vi "11_DvDt_OFF.vi"(0 "file path (IN)":path, 1 "VCE":dbl, 5 "Project #":string, 7 "Request #":string, 9 "TEST #":string, 11 "error in (no error)":errorcluster) -> (4 "file path (OUT)":path, 6 "Dv/Dt (V/us)":dbl, 8 "DONE Dv/Dt OFF":bool, 10 "OFF Region":waveform(dbl)[](graph) caption="DvDt off (V/us)", 13 "Dv (V)":dbl, 14 "Dt (ns)":dbl, 15 "error out":errorcluster)   [LabVIEW 2020]
uses:
  <vilib>/Waveform/WDTOps.llb/WDT Waveform Duration DBL.vi
  <vilib>/Waveform/WDTOps.llb/WDT Get Waveform Subset DBL.vi
  <vilib>/measure/mascope.llb/Transition Measurements 1 chan.vi
  <vilib>/measure/NI_MAPro.lvlib
panel:
  in  "Decision ?":bool
  out "Cursor b : Channel 3":dbl
  out "Cursor a : Channel 3":dbl
  in  "Cursor b : Channel 3 \nrise edge tolerance":dbl=0.1
  in  "Cursor b : Channel 3\nrise edge number":i32=1 min=1
  in  "Cursor a : Channel 3 \nrise edge tolerance":dbl=0.1
  in  "Cursor a : Channel 3\nrise edge number":i32=1 min=1
  out "Dt (us)":dbl
  out "80% Vce":dbl
  out "50% Vce":dbl
  out "measurement info (CH3 Cursor a)":T1 {"ref levels"."ref units" items=["absolute", "relative"]; "ref levels"."high ref level" format="%.2p"; "ref levels"."low ref level" format="%.2p"; "ref levels"."mid ref level" format="%.2p"; "end time" format="%.6e"; "start time" format="%.6e"}
  out "measurement info (CH3 Cursor b)":T1 {"ref levels"."ref units" items=["absolute", "relative"]; "ref levels"."high ref level" format="%.2p"; "ref levels"."low ref level" format="%.2p"; "ref levels"."mid ref level" format="%.2p"; "end time" format="%.6e"; "start time" format="%.6e"}
  in  "reference  levels (CH1 2nd Cursor)":T2={"high ref level"=90.0, "mid ref level"=50.0, "low ref level"=10.0, "ref units"=1} {"ref units" items=["absolute", "percent"]; "high ref level" format="%0.2f"; "low ref level" format="%0.2f"; "mid ref level" format="%0.2f"}
  in  "reference  levels (CH1 1st Cursor)":T2={"high ref level"=90.0, "mid ref level"=50.0, "low ref level"=10.0, "ref units"=1} {"ref units" items=["absolute", "percent"]; "high ref level" format="%0.2f"; "low ref level" format="%0.2f"; "mid ref level" format="%0.2f"}
  out "Waveform Graph":waveform(dbl)[](graph)
  # "From 50% to 80% of Peak Voltage"
  # "Default = 1"
  # "Default = 1"
  # "Default = 0.1"
  # "Default = 0.1"
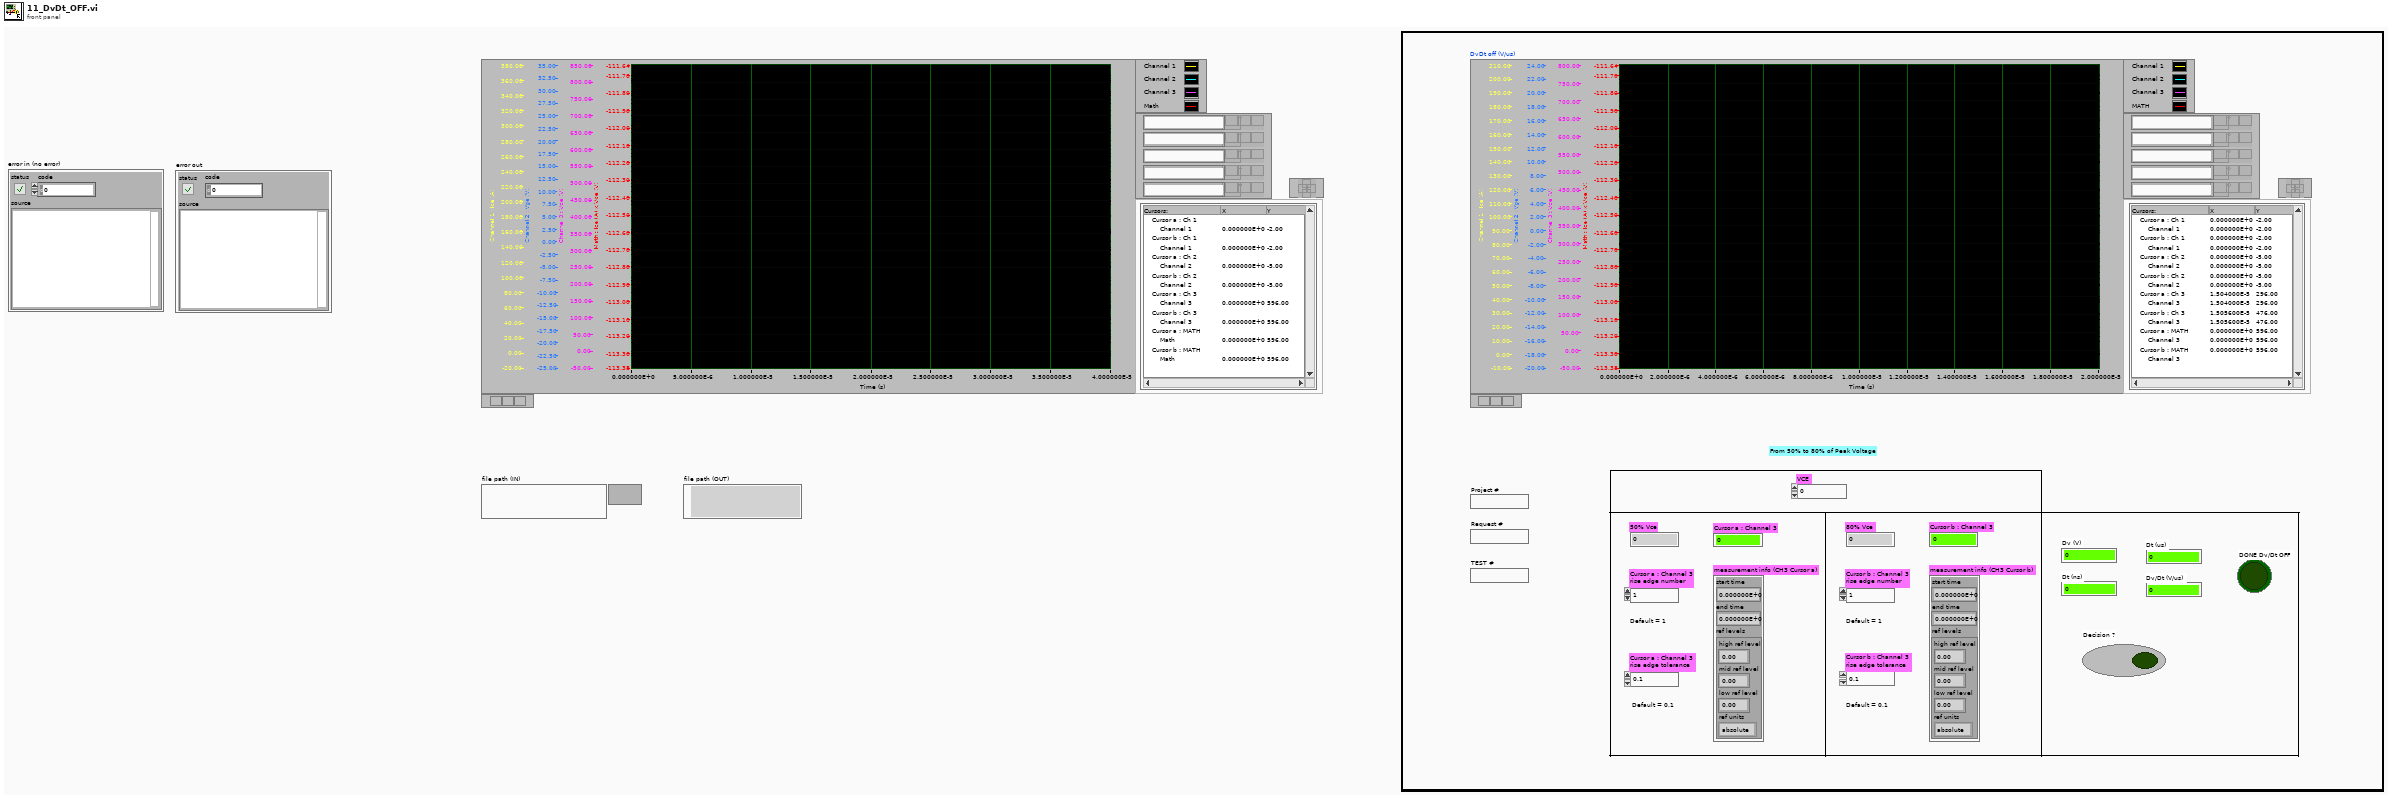
[diagram p1: front panel]
types:
  T1 = cluster{"start time":dbl, "end time":dbl, "ref levels":cluster{"high ref level":dbl, "mid ref level":dbl, "low ref level":dbl, "ref units":u16}}
  T2 = cluster{"high ref level":dbl, "mid ref level":dbl, "low ref level":dbl, "ref units":u16}
  T3 = enum32{"Invalid", "Standard", "Closed", "Hidden", "Minimized", "Maximized"}
  T4 = typedef "imagedata.ctl" = cluster{"image type":i32, "image depth":i32, "image":u8[], "mask":u8[], "colors":u32[], "Rectangle":cluster{"left":i16, "top":i16, "right":i16, "bottom":i16}}
diagram:
  w12 = 0.0 ("Dv (V)")
  w13 = errorcluster {"status"=FALSE, "code"=0, "source"=""} ("error out")
  w11 = FALSE ("DONE Tdon")
  w14 = waveform(dbl)[] [] ("Waveform Graph")
  n1 = local write "error out"(w13) -> ()
  n2 = local write "error in (no error)"(w13) -> ()
  n3 = local write "DONE Dv/Dt OFF"(w11) -> ()
  n4 = local write "Waveform Graph"(w14) -> ()
  n5 = local write "OFF Region"(w14) -> ()
  n6 = local write "Decision ?"(w11) -> ()
  n7 = local write "Cursor a : Channel 3 \nrise edge tolerance"(0.1 ("Cursor a : Channel 3 \nrise edge tolerance")) -> ()
  n8 = local write "Cursor a : Channel 3\nrise edge number"(1 ("Cursor a : Channel 3\nrise edge number")) -> ()
  n9 = local write "Cursor b : Channel 3 \nrise edge tolerance"(0.1 ("Cursor b : Channel 3 \nrise edge tolerance")) -> ()
  n10 = local write "Cursor b : Channel 3\nrise edge number"(1 ("Cursor b : Channel 3\nrise edge number")) -> ()
  n11 = local write "Dv (V)"(w12) -> ()
  n12 = local write "Dt (ns)"(w12) -> ()
  n13 = local write "Dt (us)"(w12) -> ()
  n14 = local write "Dv/Dt (V/us)"(w12) -> ()
  n15 = local write "Cursor a : Channel 3"(w12) -> ()
  n16 = local write "Cursor b : Channel 3"(w12) -> ()
  n17 = flat-sequence {
    tunnel: ["error in (no error)"] -> w6
    tunnel: ["file path (IN)"] -> w5
    tunnel: [w25] -> w9
    tunnel: [w24] -> w8
    tunnel: w6 -> [w23]
    tunnel: w5 -> [w22]
    tunnel: [w257] -> w10
    tunnel: w9 -> [w256]
    tunnel: w8 -> [w255]
    tunnel: [w255] -> w7
    tunnel: w10 -> [w270]
    tunnel: w7 -> [w271]
    frame #0 {
      n18 = control-ref of="This VI"() -> (w19:refnum<vi>)
      n19 = invoke class="VI" method="FP.Open"(reference=w19, error in="error in (no error)", "Activate"=TRUE ("Activate?"), "State"=T3."Maximized") -> (error out=w20:errorcluster)  [unwired: 1 in, 4 out]
      n20 = property class="VI"(reference=w19, error in=w20, "Front Panel.Closeable"=TRUE ("Front Panel Window:Closeable")) -> ()  [unwired: 2 out]
    }
    frame #1 {
      n21 = while {
        shift-right: [w30] -> w25
        shift-left: w23 -> [w32]
        tunnel: [w27] -> w24
        tunnel: w22 -> [w26]
        stop <- w29 stop-if-true
        n22 = flat-sequence {
          tunnel: [w58] -> w51
          tunnel: w32 -> [w63]
          tunnel: [w63] -> w31
          tunnel: w26 -> [w58]
          tunnel: w51 -> [w150]
          tunnel: [w79] -> w50
          tunnel: [w69] -> w49
          tunnel: [w65] -> w48
          tunnel: w31 -> [w156]
          tunnel: w50 -> [w199]
          tunnel: [w180] -> w47
          tunnel: w49 -> [w192]
          tunnel: [w192] -> w46
          tunnel: [w170] -> w45
          tunnel: [w169] -> w44
          tunnel: [w179] -> w43
          tunnel: [w178] -> w42
          tunnel: w48 -> [w177]
          tunnel: w47 -> [w226]
          tunnel: [w227] -> w41
          tunnel: w46 -> [w230]
          tunnel: [w230] -> w40
          tunnel: w45 -> [w229]
          tunnel: [w229] -> w39
          tunnel: w44 -> [w228]
          tunnel: [w228] -> w38
          tunnel: w43 -> [w220]
          tunnel: [w220] -> w37
          tunnel: w42 -> [w221]
          tunnel: [w221] -> w36
          tunnel: w41 -> [w231]
          tunnel: w40 -> [w244]
          tunnel: [w244] -> w35
          tunnel: w39 -> [w238]
          tunnel: w38 -> [w239]
          tunnel: w37 -> [w237]
          tunnel: w36 -> [w236]
          tunnel: [w231] -> w34
          tunnel: w35 -> [w249]
          tunnel: w34 -> [w251]
          tunnel: [w250] -> w33
          tunnel: [w249] -> w27
          frame #0 {
            w61 = 0.0 ("Dv (V)")
            w62 = FALSE ("DONE Tdon")
            w60 = waveform(dbl)[] [] ("Waveform Graph")
            n23 = local write "DONE Dv/Dt OFF"(w62) -> ()
            n24 = local write "Dv (V)"(w61) -> ()
            n25 = local write "Dt (ns)"(w61) -> ()
            n26 = local write "Dt (us)"(w61) -> ()
            n27 = local write "Dv/Dt (V/us)"(w61) -> ()
            n28 = local write "Decision ?"(w62) -> ()
            n29 = Wait (ms)(milliseconds to wait=u32 200) -> ()  [unwired: 1 out]
            n30 = local write "Cursor a : Channel 3"(w61) -> ()
            n31 = local write "Cursor b : Channel 3"(w61) -> ()
            n32 = local write "Waveform Graph"(w60) -> ()
            n33 = local write "OFF Region"(w60) -> ()
          }
          frame #1 {
            w64 = 0.0 ("start samples/time")
            w131 = u16 1 items=["Samples", "Relative Time"] ("start/duration format")
            w142 = u16 1 items=["Samples", "Relative Time"] ("start/duration format")
            w143 = u16 1 items=["Samples", "Relative Time"] ("start/duration format")
            # "Channel 1"
            # "Channel 3"
            # "Channel 2"
            # "dt"
            # "Ch2"
            # "Ch1"
            n34 = call "3_ReadDatatoWaveform.vi"("error in (no error)"=w156, "file path (IN)"=w150) -> ("error out"=w125:errorcluster, "Waveform Graph"=→"Waveform Graph":waveform(dbl)[], "file path (OUT)"=w69:path, "dt"=w151:dbl, "Ch 2 Data"=w148:dbl[], "Ch 3 Data"=w152:dbl[], "Ch 1 Data"=w149:dbl[])  [unwired: 3 in]
            n35 = To Time Stamp(1:0.0 ("number")) -> (0:w153:timestamp)
            n36 = disable-structure shown="Enabled" {
              disable-tunnel: w153 -> [w160 _]
              disable-tunnel: w151 -> [w159 _]
              disable-tunnel: w149 -> [w158 _]
              disable-tunnel: [w157 _] -> w130
              frame Enabled {
                # "Channel 1"
                n37 = Bundle By Name("Y"=w158, "dt"=w159, "t0"=w160) -> (w157:waveform(dbl))  [unwired: 1 in]
              }
              frame Disabled {
              }
            }
            n38 = disable-structure shown="Enabled" {
              disable-tunnel: w153 -> [w164 _]
              disable-tunnel: w151 -> [w163 _]
              disable-tunnel: w148 -> [w162 _]
              disable-tunnel: [w161 _] -> w129
              frame Enabled {
                # "Channel 2"
                n39 = Bundle By Name("Y"=w162, "dt"=w163, "t0"=w164) -> (w161:waveform(dbl))  [unwired: 1 in]
              }
              frame Disabled {
              }
            }
            n40 = disable-structure shown="Enabled" {
              disable-tunnel: w153 -> [w168 _]
              disable-tunnel: w151 -> [w167 _]
              disable-tunnel: w152 -> [w166 _]
              disable-tunnel: [w165 _] -> w128
              frame Enabled {
                # "Channel 3"
                n41 = Bundle By Name("Y"=w166, "dt"=w167, "t0"=w168) -> (w165:waveform(dbl))  [unwired: 1 in]
              }
              frame Disabled {
              }
            }
            n42 = call-poly <vilib>:"Waveform Duration.vi"("error in (no error)"=w125, "waveform in"=w128) -> ("error out"=w136:errorcluster, "duration"=w133:dbl, "waveform out"=w135:waveform(dbl))  [unwired: 7 in]
            n43 = call-poly <vilib>:"Waveform Duration.vi"("error in (no error)"=w125, "waveform in"=w129) -> ("error out"=w137:errorcluster, "duration"=w140:dbl, "waveform out"=w138:waveform(dbl))  [unwired: 7 in]
            n44 = call-poly <vilib>:"Waveform Duration.vi"("error in (no error)"=w125, "waveform in"=w130) -> ("error out"=w147:errorcluster, "duration"=w144:dbl, "waveform out"=w146:waveform(dbl))  [unwired: 7 in]
            n45 = Divide(x=w133, y=2.0) -> (x/y=w132:dbl)
            n46 = Divide(x=w140, y=2.0) -> (x/y=w141:dbl)
            n47 = Divide(x=w144, y=2.0) -> (x/y=w126:dbl)
            n48 = call-poly <vilib>:"Get Waveform Subset.vi"("start/duration format"=w131, "error in (no error)"=w136, "duration"=w132, "start samples/time"=w64, "waveform in"=w135) -> ("error out"=w122:errorcluster, "waveform out"=w65:waveform(dbl))  [unwired: 1 in, 2 out]
            n49 = call-poly <vilib>:"Get Waveform Subset.vi"("start/duration format"=w142, "error in (no error)"=w137, "duration"=w141, "start samples/time"=w64, "waveform in"=w138) -> ("error out"=w123:errorcluster, "waveform out"=w81:waveform(dbl))  [unwired: 1 in, 2 out]
            n50 = call-poly <vilib>:"Get Waveform Subset.vi"("start/duration format"=w143, "error in (no error)"=w147, "duration"=w126, "start samples/time"=w64, "waveform in"=w146) -> ("error out"=w124:errorcluster, "waveform out"=w80:waveform(dbl))  [unwired: 1 in, 2 out]
            n51 = Build Array(w80, w81, w65) -> (→"OFF Region":waveform(dbl)[])
            n52 = Merge Errors(w124, w123, w122) -> (w77:errorcluster)
            n53 = property on="OFF Region" class="WFGraph (strict)"(error in=w77) -> (error out=w76:errorcluster, "Width"=w75:u32)  [unwired: 1 in, 1 out]
            n54 = property on="OFF Region" class="WFGraph (strict)"(error in=w76, "Caption.Justify"=enum16{"Left", "Center", "Right"}."Left" ("Caption.Justification"), "Caption.Width"=w75, "Caption.FontBold"=TRUE ("Caption.Font:Bold"), "Caption.FontColor"=u32 16860 ("Caption.Font:Color"), "Caption.FontSize"=u32 24 ("Caption.Font:Size"), "Caption.Text"="DvDt off (V/us)") -> (error out=w71:errorcluster)  [unwired: 1 in, 1 out]
            n55 = property on="OFF Region" class="WFGraph (strict)"(error in=w71, "XScale.Offset"=w64) -> (error out=w105:errorcluster)  [unwired: 1 in, 1 out]
            n56 = property on="OFF Region" class="WFGraph (strict)"(error in=w105, "Active Cursor"=u32 0, "Cursor.Cursor X"=0.0 ("Cursor.Cursor Position:Cursor X"), "Cursor.Cursor Y"=0.0 ("Cursor.Cursor Position:Cursor Y"), "Cursor.Visible"=FALSE) -> (error out=w104:errorcluster)  [unwired: 1 in, 1 out]
            n57 = property on="OFF Region" class="WFGraph (strict)"(error in=w104, "Active Cursor"=u32 1, "Cursor.Cursor X"=0.0 ("Cursor.Cursor Position:Cursor X"), "Cursor.Cursor Y"=0.0 ("Cursor.Cursor Position:Cursor Y"), "Cursor.Visible"=FALSE) -> (error out=w103:errorcluster)  [unwired: 1 in, 1 out]
            n58 = property on="OFF Region" class="WFGraph (strict)"(error in=w103, "Active Cursor"=u32 2, "Cursor.Cursor X"=0.0 ("Cursor.Cursor Position:Cursor X"), "Cursor.Cursor Y"=0.0 ("Cursor.Cursor Position:Cursor Y"), "Cursor.Visible"=FALSE) -> (error out=w102:errorcluster)  [unwired: 1 in, 1 out]
            n59 = property on="OFF Region" class="WFGraph (strict)"(error in=w102, "Active Cursor"=u32 3, "Cursor.Cursor X"=0.0 ("Cursor.Cursor Position:Cursor X"), "Cursor.Cursor Y"=0.0 ("Cursor.Cursor Position:Cursor Y"), "Cursor.Visible"=FALSE) -> (error out=w85:errorcluster)  [unwired: 1 in, 1 out]
            n60 = property on="OFF Region" class="WFGraph (strict)"(error in=w85, "Active Cursor"=u32 4, "Cursor.Cursor X"=0.0 ("Cursor.Cursor Position:Cursor X"), "Cursor.Cursor Y"=0.0 ("Cursor.Cursor Position:Cursor Y"), "Cursor.Visible"=FALSE) -> (error out=w84:errorcluster)  [unwired: 1 in, 1 out]
            n61 = property on="OFF Region" class="WFGraph (strict)"(error in=w84, "Active Cursor"=u32 5, "Cursor.Cursor X"=0.0 ("Cursor.Cursor Position:Cursor X"), "Cursor.Cursor Y"=0.0 ("Cursor.Cursor Position:Cursor Y"), "Cursor.Visible"=FALSE) -> (error out=w83:errorcluster)  [unwired: 1 in, 1 out]
            n62 = property on="OFF Region" class="WFGraph (strict)"(error in=w83, "Active Cursor"=u32 6, "Cursor.Cursor X"=0.0 ("Cursor.Cursor Position:Cursor X"), "Cursor.Cursor Y"=0.0 ("Cursor.Cursor Position:Cursor Y"), "Cursor.Visible"=FALSE) -> (error out=w82:errorcluster)  [unwired: 1 in, 1 out]
            n63 = property on="OFF Region" class="WFGraph (strict)"(error in=w82, "Active Cursor"=u32 7, "Cursor.Cursor X"=0.0 ("Cursor.Cursor Position:Cursor X"), "Cursor.Cursor Y"=0.0 ("Cursor.Cursor Position:Cursor Y"), "Cursor.Visible"=FALSE) -> (error out=w79:errorcluster)  [unwired: 1 in, 1 out]
            n64 = call <vilib>:"Beep.vi"("use system alert? (T)"=FALSE, "duration (msec)"=u32 200, "frequency (Hz)"=u32 2000) -> ()  [unwired: 9 in]
          }
          frame #2 {
            w212 = u16 1 items=["falling", "rising"] ("polarity (rising)")
            w213 = u16 1 items=["falling", "rising"] ("polarity (rising)")
            # "XPOS"
            # "YPOS"
            # "Cursor a : Channel 1"
            # "Cursor b : Channel 1"
            # "Cursor b : Channel 1"
            # "Cursor a : Channel 1"
            # "Cursor b : Channel 1"
            # "Cursor a : Channel 3"
            # "Cursor b : Channel 1"
            # "Cursor a : Channel 3"
            # "End Time 1st Cursor"
            # "End Time 2nd Cursor"
            # "1st PARAMETER : 50% Vce"
            # "Channel 1"
            # "2nd PARAMETER : 80% Vce"
            # "Channel 1"
            n65 = Divide(x=50.0, y=100.0) -> (x/y=w219:dbl)
            n66 = Multiply(x=w219, y="VCE") -> (x*y=w187:dbl)
            "50% Vce" <- w187
            n67 = Add(x=w187, y="Cursor a : Channel 3 \nrise edge tolerance") -> (x+y=w205:dbl)
            n68 = Subtract(x=w187, y="Cursor a : Channel 3 \nrise edge tolerance") -> (x-y=w204:dbl)
            n69 = Bundle By Name(cluster="reference  levels (CH1 1st Cursor)", "high ref level"=w205, "mid ref level"=w187, "low ref level"=w204, "ref units"=u16 0) -> (w201:T2)
            n70 = call-poly <vilib>:"Transition Measurements.vi"("edge number (1)"="Cursor a : Channel 3\nrise edge number", "error in (no error)"=w199, "reference levels"=w201, "polarity (rising)"=w213, "signal in"=w177) -> ("error out"=w196:errorcluster, "measurement info"=w200:T1)  [unwired: 1 in, 4 out]
            "measurement info (CH3 Cursor a)" <- w200
            n71 = Unbundle By Name(w200) -> ("end time"=w178:dbl)
            n72 = property on="OFF Region" class="WFGraph (strict)"(error in=w196, "Active Cursor"=u32 4, "Cursor.Cursor X"=w178, "Cursor.Visible"=TRUE, "Cursor.Cursor Name Visible"=TRUE) -> (error out=w185:errorcluster)  [unwired: 1 in, 1 out]
            n73 = property on="OFF Region" class="WFGraph (strict)"(error in=w185, "Active Cursor"=u32 4) -> (error out=w183:errorcluster, "Cursor.Cursor Y"=w170:dbl)  [unwired: 1 in, 1 out]
            "Cursor a : Channel 3" <- w170
            n74 = Divide(x=80.0, y=100.0) -> (x/y=w216:dbl)
            n75 = Multiply(x=w216, y="VCE") -> (x*y=w188:dbl)
            "80% Vce" <- w188
            n76 = Add(x=w188, y="Cursor b : Channel 3 \nrise edge tolerance") -> (x+y=w211:dbl)
            n77 = Subtract(x=w188, y="Cursor b : Channel 3 \nrise edge tolerance") -> (x-y=w210:dbl)
            n78 = Bundle By Name(cluster="reference  levels (CH1 2nd Cursor)", "high ref level"=w211, "mid ref level"=w188, "low ref level"=w210, "ref units"=u16 0) -> (w207:T2)
            n79 = call-poly <vilib>:"Transition Measurements.vi"("edge number (1)"="Cursor b : Channel 3\nrise edge number", "error in (no error)"=w183, "reference levels"=w207, "polarity (rising)"=w212, "signal in"=w177) -> ("error out"=w193:errorcluster, "measurement info"=w206:T1)  [unwired: 1 in, 4 out]
            "measurement info (CH3 Cursor b)" <- w206
            n80 = Unbundle By Name(w206) -> ("end time"=w179:dbl)
            n81 = property on="OFF Region" class="WFGraph (strict)"(error in=w193, "Active Cursor"=u32 5, "Cursor.Cursor X"=w179, "Cursor.Visible"=TRUE, "Cursor.Cursor Name Visible"=TRUE) -> (error out=w181:errorcluster)  [unwired: 1 in, 1 out]
            n82 = call <vilib>:"Beep.vi"("use system alert? (T)"=FALSE, "duration (msec)"=u32 200, "frequency (Hz)"=u32 2000) -> ()  [unwired: 9 in]
            n83 = property on="OFF Region" class="WFGraph (strict)"(error in=w181, "Active Cursor"=u32 5) -> (error out=w180:errorcluster, "Cursor.Cursor Y"=w169:dbl)  [unwired: 1 in, 1 out]
            "Cursor b : Channel 3" <- w169
          }
          frame #3 {
            # "2nd Cursor"
            # "1st Cursor"
            n84 = Subtract(x=w221, y=1e-07) -> (x-y=w223:dbl)
            n85 = Add(x=w220, y=1e-07) -> (x+y=w222:dbl)
            n86 = property on="OFF Region" class="WFGraph (strict)"(error in=w226, "XScale.Minimum"=w223, "XScale.Maximum"=w222) -> (error out=w227:errorcluster)  [unwired: 1 in, 1 out]
          }
          frame #4 {
            # "us"
            # "ns"
            n87 = Subtract(x=w239, y=w238) -> (x-y=w235:dbl)
            n88 = Subtract(x=w237, y=w236) -> (x-y=w233:dbl)
            n89 = Absolute Value(x=w235) -> (abs(x)=w234:dbl)
            "Dv (V)" <- w234
            n90 = Absolute Value(x=w233) -> (abs(x)=w232:dbl)
            n91 = Multiply(x=w232, y=1000000000.0) -> (x*y=→"Dt (ns)":dbl)
            n92 = Multiply(x=w232, y=1000000.0) -> (x*y=w241:dbl)
            "Dt (us)" <- w241
            n93 = Divide(x=w234, y=w241) -> (x/y=→"Dv/Dt (V/us)":dbl)
            n94 = call <vilib>:"Beep.vi"("use system alert? (T)"=FALSE, "duration (msec)"=u32 200, "frequency (Hz)"=u32 2000) -> ()  [unwired: 9 in]
          }
          frame #5 {
            n95 = while {
              shift-right: [w252] -> w250
              shift-left: w251 -> [w252]
              stop <- "Decision ?" stop-if-true
              n96 = Wait (ms)(milliseconds to wait=u32 100) -> ()  [unwired: 1 out]
            }
          }
        }
        n97 = while {
          tunnel: [w53] -> w29
          shift-right: [w56] -> w30
          shift-left: w33 -> [w57]
          stop <- w55 stop-if-true
          n98 = Wait (ms)(milliseconds to wait=u32 100) -> ()  [unwired: 1 out]
          n99 = call "Display Message to User"("error in (no error)"=w57) -> ("error out"=w56:errorcluster, "NO"=w53:bool)  [unwired: 9 in]
          n100 = Or(x=w53, y=TRUE) -> (x .or. y?=w55:bool)
        }
        n101 = Wait (ms)(milliseconds to wait=u32 100) -> ()  [unwired: 1 out]
      }
    }
    frame #2 {
      w260 = "_"
      n102 = invoke on="OFF Region" class="WFGraph (strict)" method="Get Image"(error in=w256) -> (error out=w263:errorcluster, "image data"=w266:T4)  [unwired: 5 in, 4 out]
      n103 = Concatenate Strings("C:\\Inductive_Switching_Project\\IndSw_Image\\" ("string"), "Project #", w260, "Request #", w260, "TEST #", w260, "DvDtoff" ("string"), ".png" ("string")) -> (w267:string)
      n104 = String To Path(string=w267) -> (path=w265:path)
      n105 = call <vilib>:"Write PNG File.vi"("error in (no error)"=w263, "image data"=w266, "path to PNG file"=w265) -> ("error out"=w257:errorcluster)  [unwired: 7 in, 1 out]
      "DONE Dv/Dt OFF" <- TRUE ("DONE Di/Dt ON")
    }
    frame #3 {
      n106 = disable-structure shown="Enabled" {
        disable-tunnel: w270 -> [w272 _]
        frame Enabled {
          n107 = control-ref of="This VI"() -> (w273:refnum<vi>)
          n108 = invoke class="VI" method="FP.Close"(reference=w273, error in=w272) -> ()  [unwired: 1 in, 3 out]
        }
        frame Disabled {
        }
      }
      "error out" <- w270
      "file path (OUT)" <- w271
    }
  }
